vi "Decode Schedule Message.vi"(8 "error in (no error)":errorcluster, 10 "Schedule message":T1, 11 "Tamer in":refnum<class "Tamer.lvclass">) -> (0 "error out":errorcluster, 3 "Tamer out":refnum<class "Tamer.lvclass">)   [LabVIEW 2020, in "Tamer.lvlib" / "Tamer.lvclass"]
uses:
  Tamer.lvclass
  Run Utilities/TypeDefs/Messages/Schedule Message - Standard.ctl
  Run Utilities/Schedule/Schedule.lvclass
  Tamer.lvclass/Tamer.ctl
  Run Utilities/TypeDefs/Synchronize FPGA Cluster.ctl
  Run Utilities/TypeDefs/Monkey Status.ctl
  Run Utilities/Run Utilities.lvlib
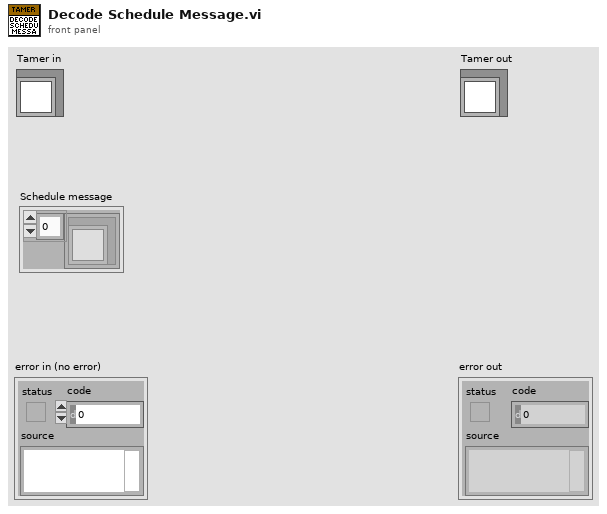
[diagram p1: front panel]
types:
  T1 = typedef "TALOS.lvlib/Run Utilities.lvlib/Schedule Message - Standard.ctl" = cluster{"Schedules":refnum<class "Schedule.lvclass">[]}
  T2 = typedef "TALOS.lvlib/Run Utilities.lvlib/Monkey Status.ctl" = enum16{"Init", "Paused", "Ongoing", "Stopped", "Finished (no errors)", "Finished (with errors)"}
  T3 = typedef "TALOS.lvlib/Run Utilities.lvlib/Synchronize FPGA Cluster.ctl" = cluster{"Status":bool, "FPGA Name":string}
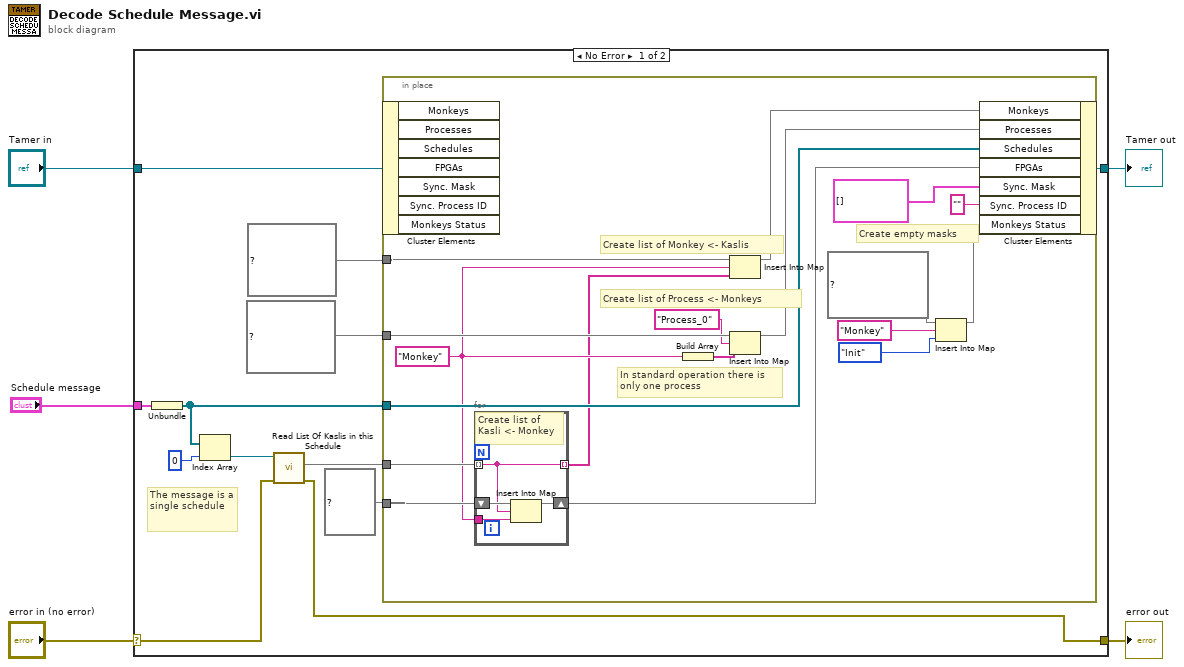
[diagram p0: block diagram]
diagram:
  n1 = case shown="No Error" "error in (no error)" {
    selector: "error in (no error)" -> [w15 w41]
    tunnel: [w6 w41] -> w4
    tunnel: [w7 w40] -> w2
    tunnel: "Tamer in" -> [w12 w40]
    tunnel: "Schedule message" -> [w10 _]
    frame No Error {
      # "The message is a single schedule"
      n2 = Unbundle(w10) -> ("Schedules"=w11:refnum<class "Schedule.lvclass">[])
      n3 = Index Array(array=w11, index=0) -> (element=w16:refnum<class "Schedule.lvclass">)
      n4 = call-dynamic "Read List Of Kaslis in this Schedule.vi"("error in (no error)"=w15, "Schedule in"=w16) -> ("error out"=w6:errorcluster, "List of FPGAs"=w14:set{string})  [unwired: 7 in, 1 out]
      n5 = in-place {
        in-place-border: w14 -> [w32]
        in-place-border: map{string, string[]} {} ("Monkeys") -> [w35]
        in-place-border: w11 -> [w30]
        in-place-border: map{string, string} {} ("Kaslis") -> [w33]
        in-place-border: map{string, string[]} {} ("Processes") -> [w29]
        w25 = "Monkey" ("key")
        # "Create empty masks"
        # "In standard operation there is only one process"
        # "Create list of Process <- Monkeys"
        # "Create list of Monkey <- Kaslis"
        n6 = in-place-cluster #1(w12) -> ()  [unwired: 7 out]
        n7 = for {
          tunnel: w32 -> [w36] mode=indexing
          shift-right: [w38] -> w31
          shift-left: w33 -> [w39]
          tunnel: w25 -> [w37]
          tunnel: [w36] -> w18 mode=indexing
          # "Create list of Kasli <- Monkey"
          n8 = Insert Into Map(map in=w39, key=w36, value=w37) -> (map out=w38:map{string, string})  [unwired: 2 out]
        }
        n9 = Build Array(w25) -> (w26:string[])
        n10 = Insert Into Map(map in=w35, key=w25, value=w18) -> (map out=w34:map{string, string[]})  [unwired: 2 out]
        n11 = Insert Into Map(map in=w29, key="Process_0", value=w26) -> (map out=w27:map{string, string[]})  [unwired: 2 out]
        n12 = Insert Into Map(map in=map{string, T2} {} ("Monkeys Status"), key="Monkey", value=Monkey_Status."Init") -> (map out=w22:map{string, T2})  [unwired: 2 out]
        n13 = in-place-cluster #1("Monkeys"=w34, "Processes"=w27, "Schedules"=w30, "FPGAs"=w31, "Sync. Mask"=T3[] [] ("Synchronize Mask"), "Sync. Process ID"="" ("Parallel Process ID"), "Monkeys Status"=w22) -> (w7:refnum<class "Tamer.lvclass">)
      }
    }
    frame Error {
    }
  }
  "error out" <- w4
  "Tamer out" <- w2
